vi "Motor_Excel_to_Array(OK).vi"() -> ()   [LabVIEW 2023]
uses:
  <vilib>/addons/_office/excel.llb/Excel Get Data ([dbl]).vi
  <vilib>/Utility/NIReport.llb/NI_report.lvclass
  <vilib>/Utility/NIReport.llb/Excel/NI_Excel.lvclass
  <vilib>/addons/_office/NI_ReportGenerationToolkit.lvlib
panel:
  in  "Cal_Max_Speed":enum32{"手動輸入 Selection 1", "參考 Table"}(radio)
  in  "Stop":bool
  in  "Tab Control":enum32{"Graph", "Array", "Vehicle", "Vehicle 2"}(tab)
  out "slope_value_(%)":dbl
  out "Road&Motor":cluster{"data":dbl[], "data":dbl[]}[](graph)
  out "Motor Max Torque":T1(graph)={"array type (2D Dbl)"=[0.0, 5.0, 10.0, 15.0, 20.0, 25.0, 30.0, 35.0, 40.0, 45.0, 50.0, 55.0, 60.0, 65.0, 70.0, 75.0, 80.0, 85.0, 90.0, 95.0, 100.0, 105.0, 110.0, 115.0, 120.0, 125.0, 130.0, 135.0, 140.0, 145.0, 150.0, 155.0, 160.0, 165.0, 170.0, 175.0, 180.0, 185.0, 190.0, 195.0, 200.0, 205.0, 210.0, 215.0, 220.0, 225.0, 230.0, 235.0, 240.0, 245.0], "array type (2D Dbl)"=[7.64, 4.95, 6.83, 9.7, 4.25, 5.21, 3.69, 9.63, 7.28, 4.87, 6.61, 3.48, 3.51, 5.43, 7.79, 2.74, 3.77, 9.97, 2.54, 5.19, 9.7, 5.12, 1.95, 1.46, 2.93, 2.02, 4.5, 5.86, 6.09, 5.11, 1.22, 8.82, 1.81, 7.21, 5.19, 4.2, 7.97, 6.75, 2.71, 3.86, 1.49, 3.44, 5.75, 5.05, 3.16, 8.68, 8.7, 4.07, 5.28, 3.4]}
  out "Motor Power Curve":T1(graph)={"array type (2D Dbl)"=[0.0, 5.0, 10.0, 15.0, 20.0, 25.0, 30.0, 35.0, 40.0, 45.0, 50.0, 55.0, 60.0, 65.0, 70.0, 75.0, 80.0, 85.0, 90.0, 95.0, 100.0, 105.0, 110.0, 115.0, 120.0, 125.0, 130.0, 135.0, 140.0, 145.0, 150.0, 155.0, 160.0, 165.0, 170.0, 175.0, 180.0, 185.0, 190.0, 195.0, 200.0, 205.0, 210.0, 215.0, 220.0, 225.0, 230.0, 235.0, 240.0, 245.0], "array type (2D Dbl)"=[7.64, 4.95, 6.83, 9.7, 4.25, 5.21, 3.69, 9.63, 7.28, 4.87, 6.61, 3.48, 3.51, 5.43, 7.79, 2.74, 3.77, 9.97, 2.54, 5.19, 9.7, 5.12, 1.95, 1.46, 2.93, 2.02, 4.5, 5.86, 6.09, 5.11, 1.22, 8.82, 1.81, 7.21, 5.19, 4.2, 7.97, 6.75, 2.71, 3.86, 1.49, 3.44, 5.75, 5.05, 3.16, 8.68, 8.7, 4.07, 5.28, 3.4]}
  in  "Road_Slope_(%)":sgl(slide) min=0 max=20 step=1 scale=0.0..20.0
  out "Tire_Torque Array(kph_Nm)":dbl[][](array[numeric]) format="%#.1f"
  out "Motor_Torque_Array (rpm_Nm)":dbl[][](array[numeric])
  in  "window state (normal)":T2(ring)=enum."normal"
  in  "report type":T3(ring)=enum."Excel"
  out "Vehicle_speed_(m/s)":dbl[](array[numeric])
  out "Vehicle_speed_(km/h)":dbl[](array[numeric])
  out "Road_Resistance_Array (kph_Nm)":dbl[][](array[numeric]) format="%#.1f"
  out "Road_Load 1 (Aero)":dbl[](array[numeric])
  out "Road_Load 2 (Roll)":dbl=0.7
  out "Road_Load_3(slope)":dbl=0.7
  in  "Trie_HWRatio_(%)":dbl=75.0
  out "Front_Area(m^2)":dbl
  out "Tire_Radius(m)":dbl=0.3835
  in  "Mass_AddFactor_(-)":dbl=1.04
  in  "Tire_Diameter_ (in)":dbl=17.5
  in  "Tire_Height_(mm)":dbl=215.0
  out "Trie Skip coefficient(-)":dbl=0.03
  in  "Reducer_Ratio_(-)":dbl=5.13
  out "rolling friction_coefficient_(-)":dbl=0.01
  out "Airdensity(kg/m^3)":dbl=1.225
  out "Graviational_constant_(m/s^2)":dbl=9.81
  out "areo_dynamic_coefficient_(-)":dbl=0.7
  in  "Powertrain_eff_(%)":dbl=85.0
  in  "Vehicle_FullLoad_(kg)":dbl=9900.0
  in  "Vehicle_width_(m)":dbl=2.3
  in  "Vehicle_Height_m)":dbl=3.0
  in  "Front_Area_constant(-)":dbl=1.0
  out "Max slope_angle_(deg)":dbl format="%.1f"
  out "Max slope_value_(%)":dbl format="%.1f"
  out "Vehicle_Max_speed_(kph)":dbl format="%.2f"
  in  "Torque _(Nm) @ Max_Motor_speed":dbl=500.0
  in  "Max_Motor_speed (rpm)":dbl=4000.0
  out "Vehicle_Max_speed":dbl format="%.2f"
  out "Road_Loading_Torque":dbl format="%.2f"
  out "Vehicle_Torque_Max_speed":dbl format="%.2f"
  out "Motor_Max_Torque(Nm)":dbl format="%.2f"
  in  "Motor _Max Torque (Nm)":dbl=2000.0
  in  "Motor_speed @ Max Torque (rpm)":dbl=1000.0
  # "檢查馬達最大扭力(Nm)"
  # "檢查馬達最大轉速 nmax (rpm)與扭力(Nm)"
  # "極速(km/hr)"
  # "最大爬坡度"
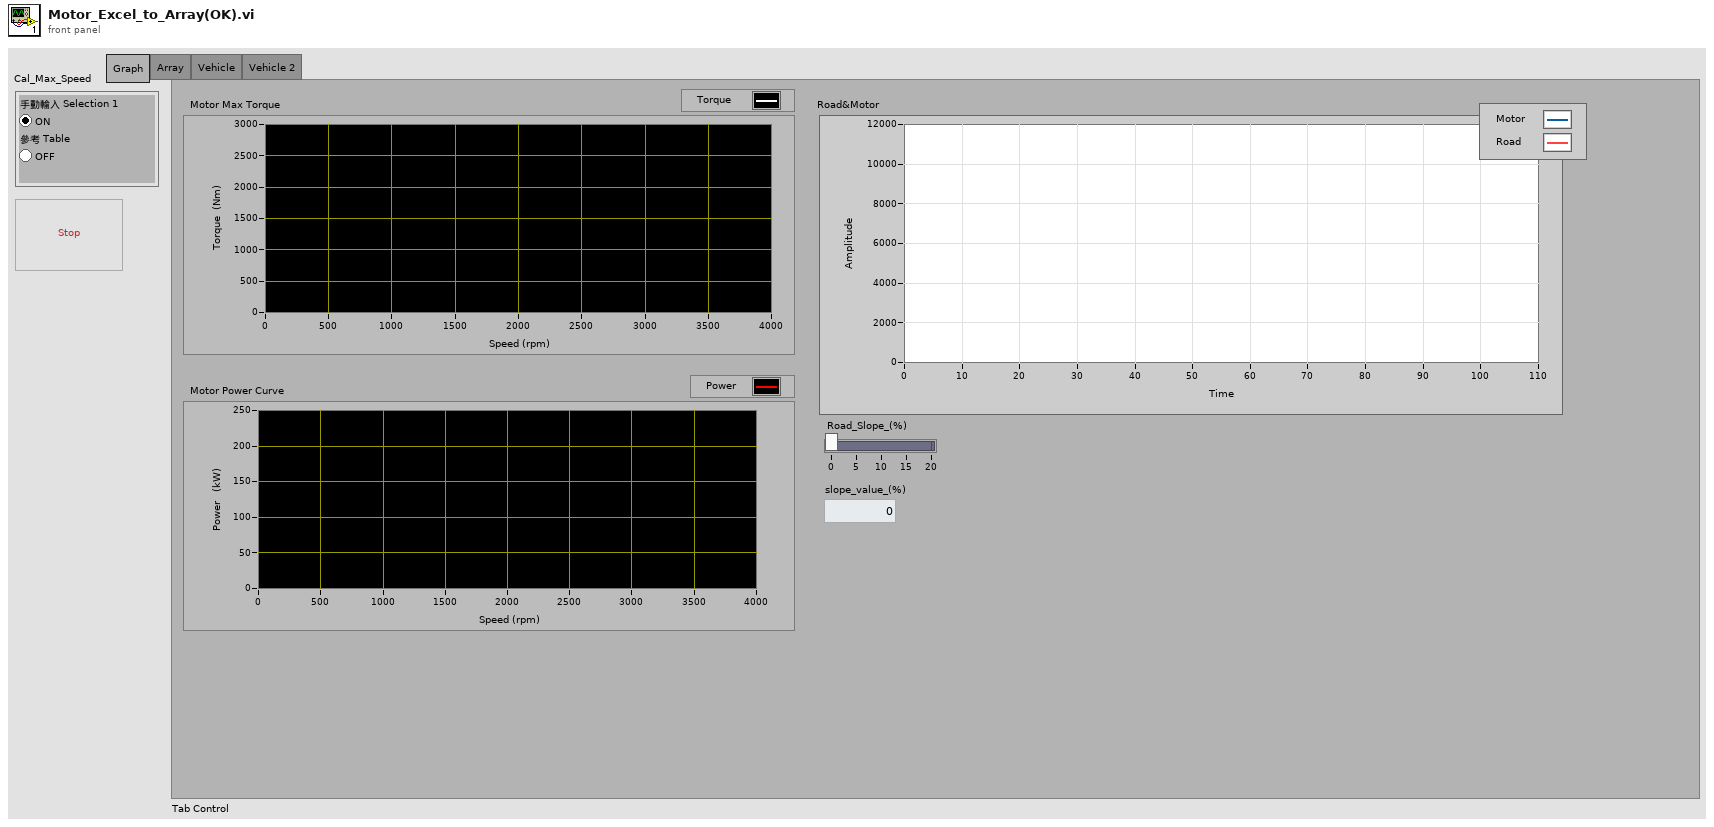
[diagram p1: front panel]
types:
  T1 = cluster{"array type (2D Dbl)":dbl[], "array type (2D Dbl)":dbl[]}
  T2 = enum16{"maximized", "minimized", "normal", "no change"}
  T3 = enum16{"Standard Report", "HTML", "Word", "Excel"}
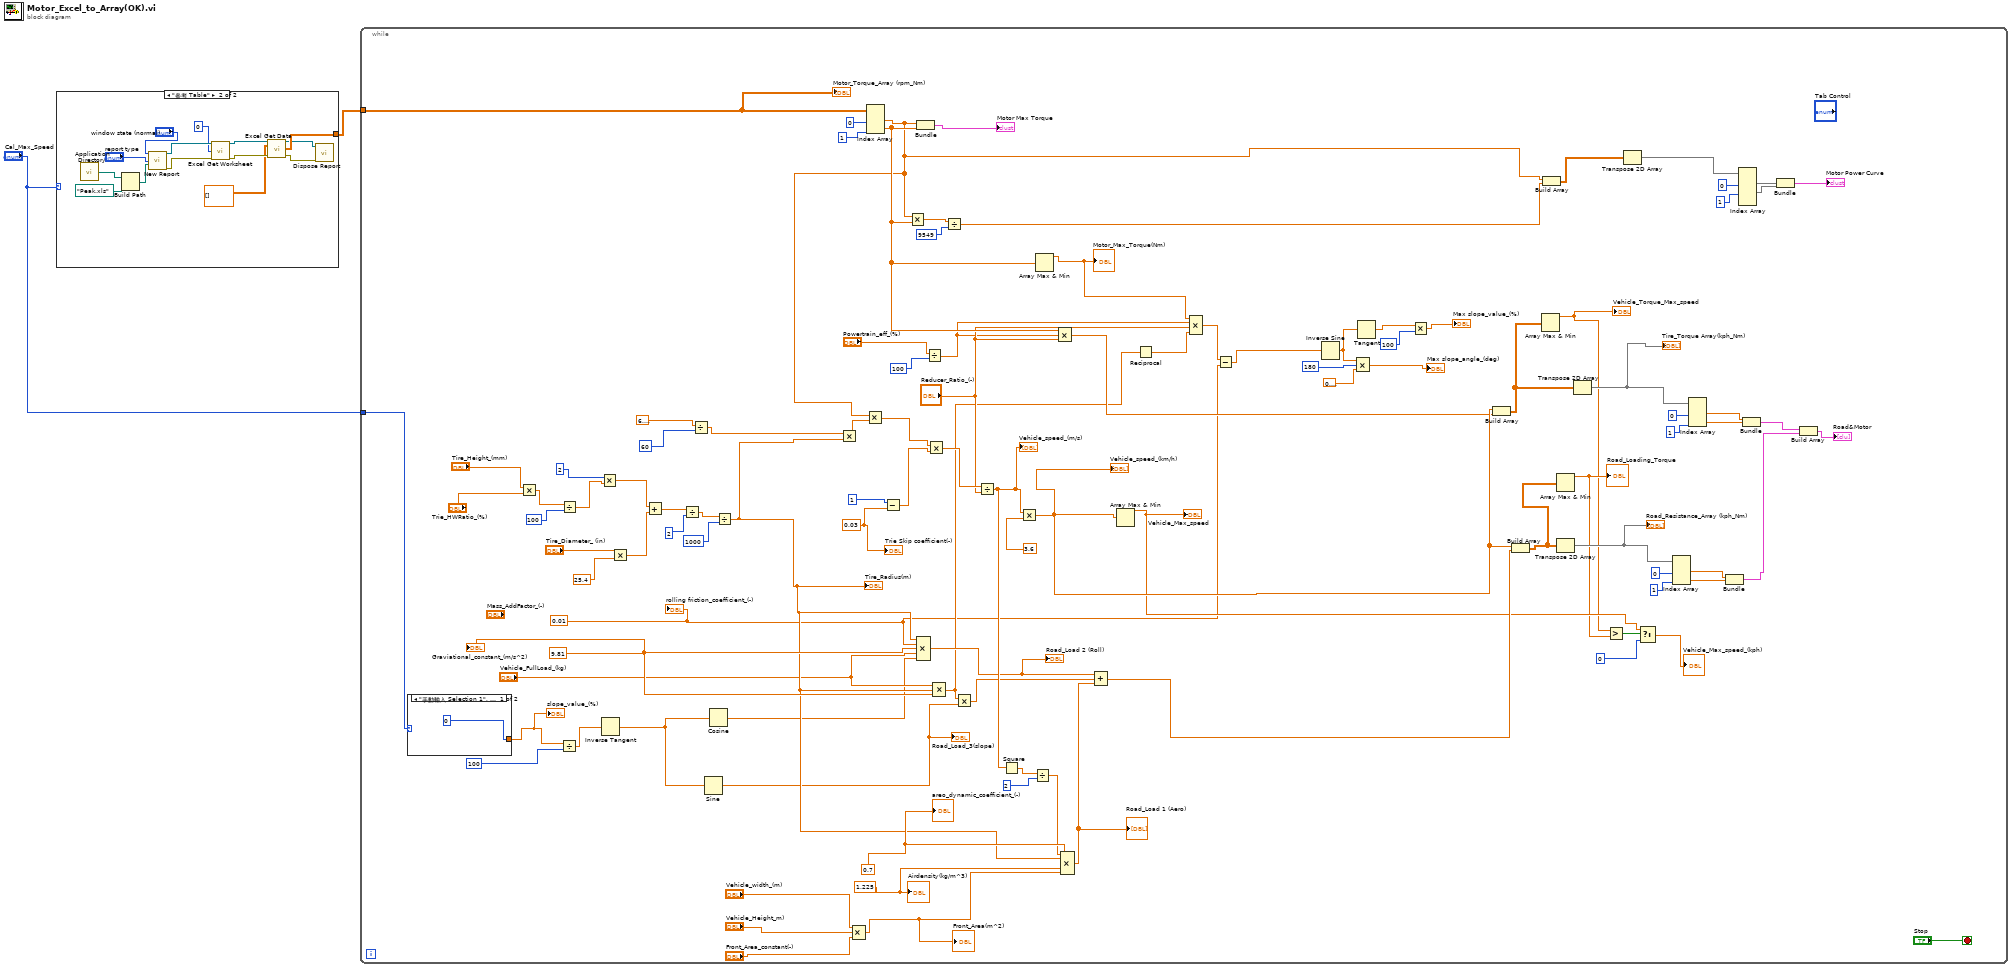
[diagram p0: block diagram]
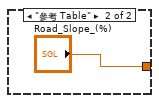
[diagram p2: hidden frame]
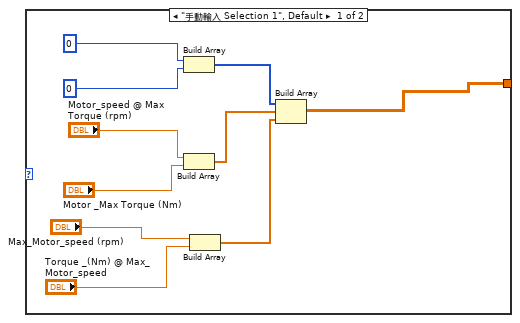
[diagram p3: hidden frame]
diagram:
  n1 = case shown="\"參考 Table\"" "Cal_Max_Speed" {
    tunnel: [w7 w21] -> w2
    frame "手動輸入 Selection 1", Default {
      n2 = Build Array(0, 0) -> (w8:i32[])
      n3 = Build Array("Motor_speed @ Max Torque (rpm)", "Motor _Max Torque (Nm)") -> (w3:dbl[])
      n4 = Build Array("Max_Motor_speed (rpm)", "Torque _(Nm) @ Max_Motor_speed") -> (w6:dbl[])
      n5 = Build Array(w8, w3, w6) -> (w7:dbl[][])
    }
    frame "參考 Table" {
      n6 = call <vilib>:"Application Directory.vi"() -> ("Application Directory"=w15:path)
      n7 = Build Path(base path=w15, name or relative path=path "Peak.xls") -> (appended path=w13:path)
      n8 = call <vilib>:"New Report.vi"("window state (normal)"="window state (normal)", "report type"="report type", "template (empty)"=w13) -> ("report out"=w25:refnum<class "NI_report.lvclass">, "error out"=w26:errorcluster)  [unwired: 11 in]
      n9 = call <vilib>:"Excel Get Worksheet.vi"("report in"=w25, "worksheet index (0)"=0, "error in (no error)"=w26) -> ("report out"=w24:refnum<class "NI_report.lvclass">, "error out"=w23:errorcluster)  [unwired: 11 in]
      n10 = call-poly <vilib>:"Excel Get Data.vi"("report in"=w24, "data type"=dbl[][] [], "error in (no error)"=w23) -> ("report out"=w17:refnum<class "NI_report.lvclass">, "data"=w21:dbl[][], "error out"=w16:errorcluster)  [unwired: 10 in]
      n11 = call-dynamic "Dispose Report.vi"("report in"=w17, "error in (no error)"=w16) -> ()  [unwired: 13 in, 1 out]
    }
  }
  n12 = while {
    tunnel: w2 -> [w123]
    tunnel: "Cal_Max_Speed" -> [w122]
    stop <- "Stop" stop-if-true
    w89 = 0.7
    w66 = 0.01
    w88 = 1.225
    w80 = 9.81
    w97 = 0.03
    n13 = case shown="\"手動輸入 Selection 1\", Default" w122 {
      tunnel: [0 "Road_Slope_(%)"] -> w27
      frame "手動輸入 Selection 1", Default {
      }
      frame "參考 Table" {
      }
    }
    "slope_value_(%)" <- w27
    n14 = Multiply(x="Tire_Height_(mm)", y="Trie_HWRatio_(%)") -> (x*y=w111:dbl)
    n15 = Divide(x=w27, y=100) -> (x/y=w76:sgl)
    n16 = Divide(x=w111, y=100) -> (x/y=w106:dbl)
    n17 = Multiply(x=2, y=w106) -> (x*y=w105:dbl)
    n18 = Inverse Tangent(1:w76) -> (0:w77:sgl)
    n19 = Multiply(x="Tire_Diameter_ (in)", y=25.4) -> (x*y=w104:dbl)
    n20 = Add(x=w105, y=w104) -> (x+y=w101:dbl)
    n21 = Divide(x=w101, y=2) -> (x/y=w99:dbl)
    n22 = Divide(x=6.283185307179586, y=60) -> (x/y=w114:dbl)
    n23 = Sine(x=w77) -> (sin(x)=w62:sgl)
    "Road_Load_3(slope)" <- w62
    n24 = Cosine(x=w77) -> (cos(x)=w70:sgl)
    n25 = Divide(x=w99, y=1000) -> (x/y=w78:dbl)
    "Tire_Radius(m)" <- w78
    n26 = Multiply(x=w114, y=w78) -> (x*y=w103:dbl)
    n27 = Compound Arithmetic op=MULTIPLY("Vehicle_width_(m)", "Vehicle_Height_m)", "Front_Area_constant(-)") -> (w84:dbl)
    "Front_Area(m^2)" <- w84
    n28 = Index Array "Index Array"(array=w123, index (col) #1=0 ("disabled index (col)"), index (col) #2=1 ("index (col)")) -> (element #1=w129:dbl[], element #2=w131:dbl[])  [unwired: 2 in]
    n29 = Multiply(x=w129, y=w103) -> (x*y=w95:dbl[])
    n30 = Subtract(x=1, y=w97) -> (x-y=w96:dbl)
    n31 = Multiply(x=w129, y=w131) -> (x*y=w117:dbl[])
    n32 = Bundle "Bundle"("data"=w129, "data"=w131) -> (→"Motor Max Torque":cluster{"data":dbl[], "data":dbl[]})  [unwired: 1 in]
    n33 = Compound Arithmetic op=MULTIPLY(w78, w66, w80, "Vehicle_FullLoad_(kg)", w70) -> (w81:dbl)
    "Road_Load 2 (Roll)" <- w81
    n34 = Divide(x="Powertrain_eff_(%)", y=100) -> (x/y=w64:dbl)
    n35 = Multiply(x=w95, y=w96) -> (x*y=w94:dbl[])
    n36 = Compound Arithmetic op=MULTIPLY("Vehicle_FullLoad_(kg)", w78, w80) -> (w68:dbl)
    n37 = Divide(x=w117, y=9549) -> (x/y=w130:dbl[])
    n38 = Multiply(x=w68, y=w62) -> (x*y=w69:dbl)
    n39 = Divide(x=w94, y="Reducer_Ratio_(-)") -> (x/y=w92:dbl[])
    "Vehicle_speed_(m/s)" <- w92
    n40 = Square(x=w92) -> (x^2=w90:dbl[])
    n41 = Multiply(x=w92, y=3.6) -> (x*y=w128:dbl[])
    "Vehicle_speed_(km/h)" <- w128
    n42 = Divide(x=w90, y=2) -> (x/y=w79:dbl[])
    n43 = Array Max & Min(array=w131) -> (max value=w73:dbl)  [unwired: 3 out]
    "Motor_Max_Torque(Nm)" <- w73
    n44 = Compound Arithmetic op=MULTIPLY(w131, w64, "Reducer_Ratio_(-)") -> (w127:dbl[])
    n45 = Compound Arithmetic op=MULTIPLY(w79, w78, w89, w88, w84) -> (w82:dbl[])
    "Road_Load 1 (Aero)" <- w82
    n46 = Compound Arithmetic op=ADD(w81, w69, w82) -> (w126:dbl[])
    n47 = Array Max & Min(array=w128) -> (max value=w125:dbl)  [unwired: 3 out]
    "Vehicle_Max_speed" <- w125
    n48 = Reciprocal(x=w68) -> (1/x=w67:dbl)
    n49 = Compound Arithmetic op=MULTIPLY(w73, w64, "Reducer_Ratio_(-)", w67) -> (w65:dbl)
    n50 = Subtract(x=w65, y=w66) -> (x-y=w124:dbl)
    n51 = Inverse Sine(1:w124) -> (0:w36:dbl)
    n52 = Compound Arithmetic op=MULTIPLY(w36, 180, 0.3183098861837907) -> (→"Max slope_angle_(deg)":dbl)
    n53 = Tangent(1:w36) -> (0:w34:dbl)
    n54 = Multiply(x=w34, y=100) -> (x*y=→"Max slope_value_(%)":dbl)
    n55 = Build Array(w128, w127) -> (w44:dbl[][])
    n56 = Build Array(w128, w126) -> (w45:dbl[][])
    n57 = Array Max & Min(array=w44) -> (max value=w41:dbl)  [unwired: 3 out]
    "Vehicle_Torque_Max_speed" <- w41
    n58 = Build Array(w129, w130) -> (w56:dbl[][])
    n59 = Array Max & Min(array=w45) -> (max value=w42:dbl)  [unwired: 3 out]
    "Road_Loading_Torque" <- w42
    n60 = Transpose 2D Array(2D array=w45) -> (transposed array=w46:dbl[][])
    "Road_Resistance_Array (kph_Nm)" <- w46
    n61 = Transpose 2D Array(2D array=w44) -> (transposed array=w51:dbl[][])
    "Tire_Torque Array(kph_Nm)" <- w51
    n62 = Greater?(x=w41, y=w42) -> (0:w40:bool)
    n63 = Transpose 2D Array(2D array=w56) -> (transposed array=w61:dbl[][])
    n64 = Select(t=w125, s=w40, f=0 ("disabled index (col)")) -> (s? t:f=→"Vehicle_Max_speed_(kph)":dbl)
    n65 = Index Array "Index Array"(array=w46, index (col) #1=0 ("disabled index (col)"), index (col) #2=1 ("index (col)")) -> (element #1=w48:dbl[], element #2=w47:dbl[])  [unwired: 2 in]
    n66 = Index Array "Index Array"(array=w51, index (col) #1=0 ("disabled index (col)"), index (col) #2=1 ("index (col)")) -> (element #1=w53:dbl[], element #2=w52:dbl[])  [unwired: 2 in]
    n67 = Bundle "Bundle"(w48, w47) -> (w29:cluster{dbl[], dbl[]})  [unwired: 1 in]
    n68 = Index Array "Index Array"(array=w61, index (col) #1=0 ("disabled index (col)"), index (col) #2=1 ("index (col)")) -> (element #1=w58:dbl[], element #2=w57:dbl[])  [unwired: 4 in, 1 out]
    n69 = Bundle "Bundle"(w53, w52) -> (w28:cluster{dbl[], dbl[]})  [unwired: 1 in]
    n70 = Bundle "Bundle"(w58, w57) -> (→"Motor Power Curve":cluster{dbl[], dbl[]})  [unwired: 1 in]
    n71 = Build Array(w28, w29) -> (→"Road&Motor":cluster{dbl[], dbl[]}[])
    "Motor_Torque_Array (rpm_Nm)" <- w123
    "Trie Skip coefficient(-)" <- w97
    "Graviational_constant_(m/s^2)" <- w80
    "Airdensity(kg/m^3)" <- w88
    "rolling friction_coefficient_(-)" <- w66
    "areo_dynamic_coefficient_(-)" <- w89
  }
